vi "Rotronic_monitor.vi"(0 "VISA resource name":refnum<visa-resource-name>="COM1", 1 "baud rate":u32=9600, 2 "data bits":u16=8 min=5 max=8 step=1, 3 "parity":u16(ring) items=["None", "Odd", "Even", "Mark", "Space"], 4 "stop bits":u16(ring)=10 items=["1.0"=10, "1.5"=15, "2.0"=20], 5 "write":bool=TRUE, 6 "read":bool=TRUE, 7 "flow control":u16(ring) items=["None"=0, "XON/XOFF"=1, "RTS/CTS"=2, "DTR/DSR"=4], 8 "string to write":string="*IDN?\r\n") -> (9 "read string":string, 10 "bytes read":u32)   [LabVIEW 2019]
doc: "The Basic Serial Read and Write example performs a Serial Port Read, a Serial Port Write, or a combination of these actions. The user selects the actions (read or write) on the front panel. If both are selected, the VI will write the data first, read data, and then close the VISA session that is opened to the port. This VI will wait until the specified number of bytes is received at the port. Only the number of bytes specified will be read.\n\nINSTRUCTIONS:\n1) Select the serial resource and configuration parameters (baud rate, data bits, parity, stop bits, flow control).\n2) Select the operations to be performed. \n3) Connect the serial port to your device. If no device is available, perform a loopback test by doing one of the following. Short pins 2 and 3 on a RS-232 cable or short pin 4 to pin 8 and pin 5 to pin 9 on a RS-485/422 cable. \n4) Run the VI to see the data read. (The \"read string\" will match the \"string to write\" if a loopback test was performed.)\n\nNote: The parameters set for the serial port must match the parameters of the connected instrument or device. In this example, the bytes to read parameter specifies the number of bytes that the serial port reads. If there were more bytes at the port than the number specified in bytes to read, those bytes would not be read. Also, if you specify to read more bytes than the number of bytes actually read, you might receive a timeout error message.\n\nOn the block diagram, the Configure Serial Port VI sets the configuration parameters. The front panel displays the controls used to configure the basic parameters, such as baud rate, data bits, and parity. Constants configure the other parameters the user probably does not need set. After the VISA Configure Serial Port VI opens the VISA session and configures the port, the VI passes the VISA resource name to other VIs that perform operations on that VISA resource. The VISA Write function sends a command to the serial device and the VISA Read function returns data based on the command. The VISA Close function then closes the reference to the serial device. It is important to close the reference; otherwise communication through with that port through protocols other than VISA might not be possible."
uses:
  <vilib>/Instr/_visa.llb/VISA Configure Serial Port (Instr).vi
panel:
  out "N2 temperature > dew point":bool
  in  "File Path Control":path
  out "Last Line":string[](array[string])
  in  "Quit":bool
  in  "delay before read (ms)":u32=500
  # "Select the serial resource and the operations (Read, Write, or both) to be performed.  If both are selected, the VI will write the data first, read data and then close the VISA session that is opened to the port.  This VI will wait until the specified number of bytes is received at the port. Only the number of bytes specified will be read."
  # "For additional information select File >> VI Properties >> Documentation"
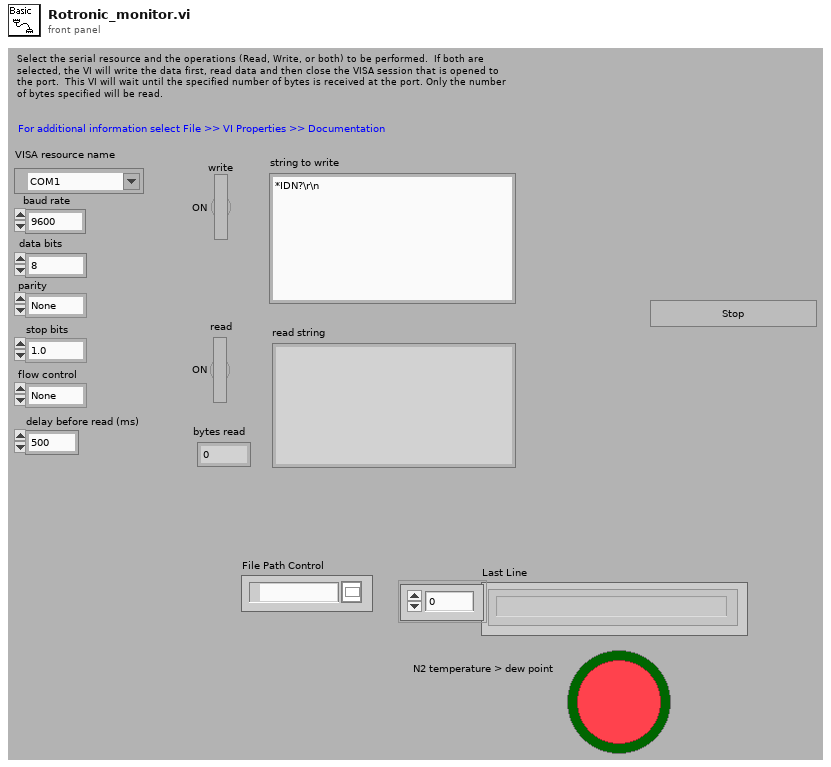
[diagram p1: front panel]
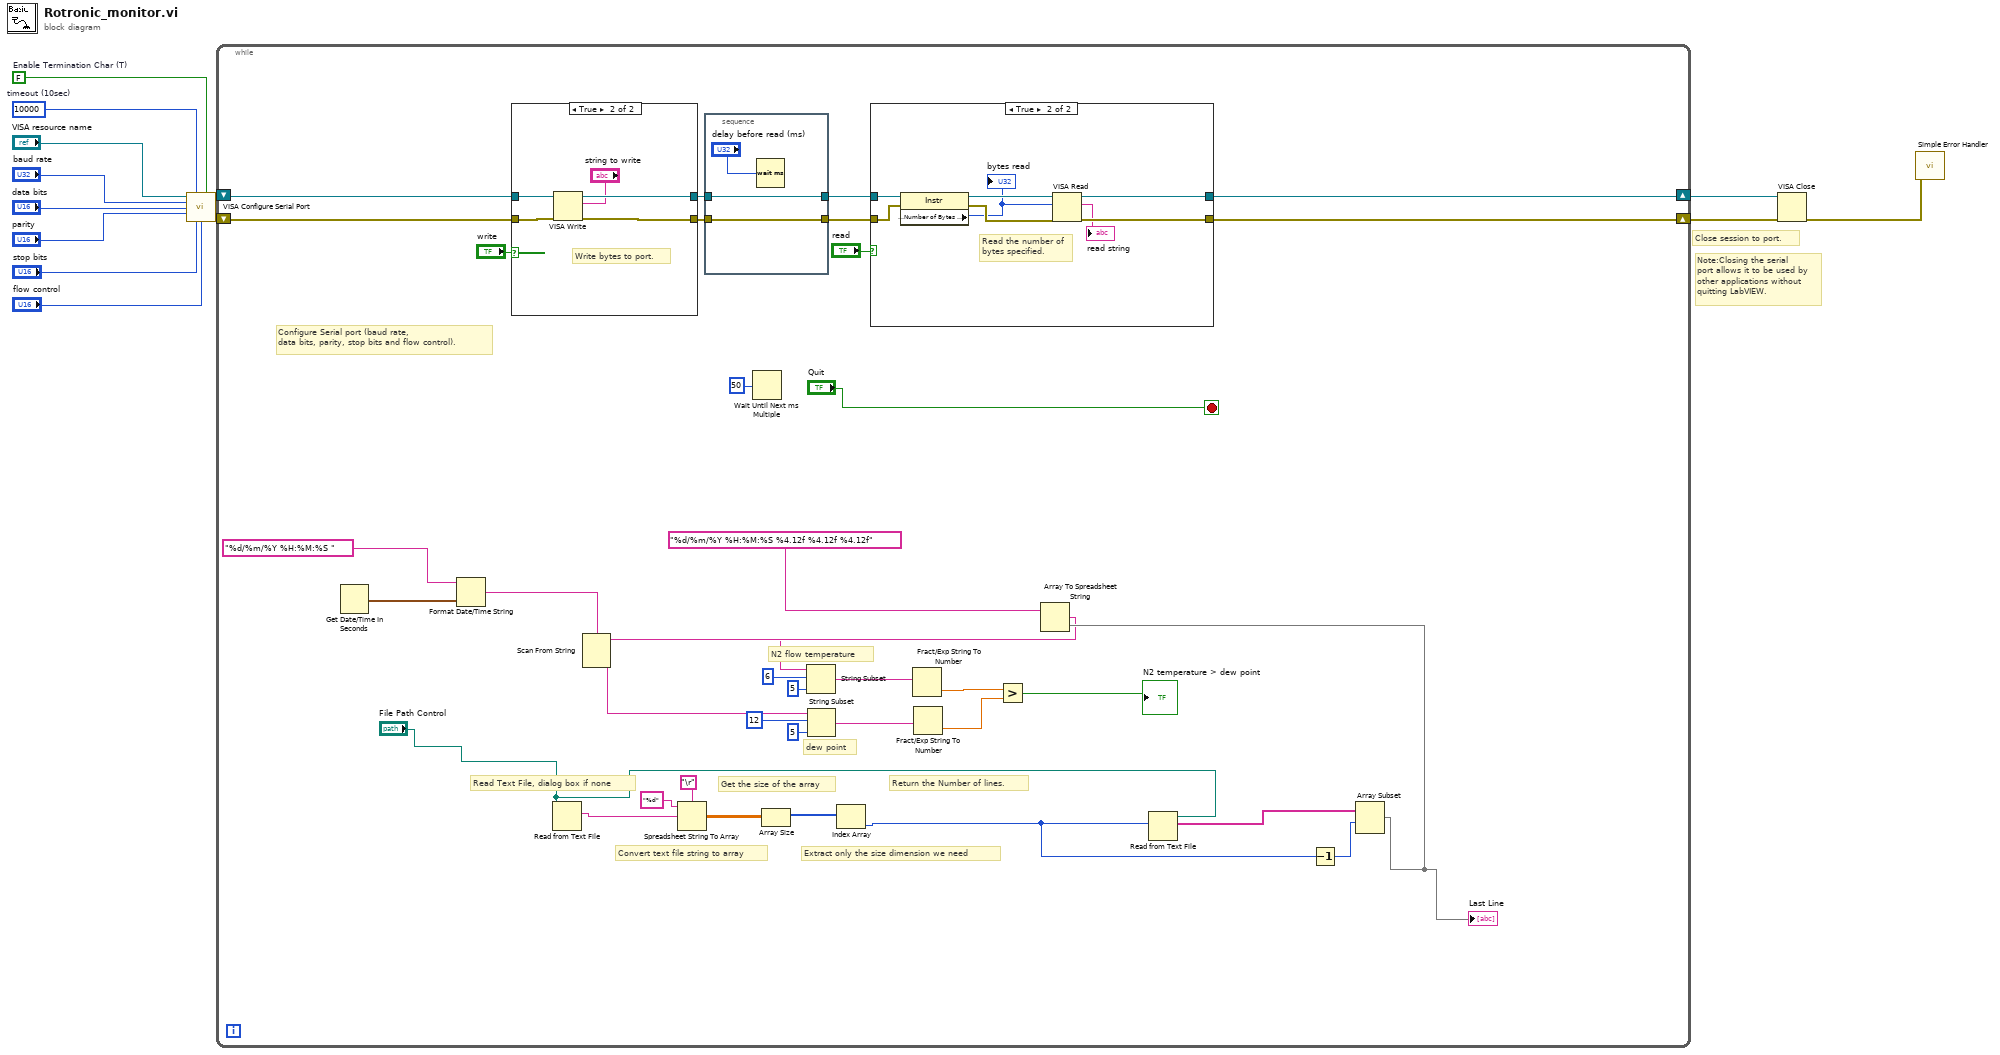
[diagram p0: block diagram]
diagram:
  w4 = FALSE  # Enable Termination Char (T)
  w5 = u32 10000  # timeout (10sec)
  # "Note:Closing the serial port allows it to be used by other applications without\nquitting LabVIEW."
  # "Close session to port."
  n1 = call-poly "VISA Configure Serial Port"("VISA resource name"="VISA resource name", "timeout (10sec)"=w5, "Enable Termination\nChar (T)"=w4, "baud rate (9600)"="baud rate", "data bits (8)"="data bits", "parity (0:none)"="parity", "stop bits (10: 1 bit)"="stop bits", "flow control (0:none)"="flow control") -> ("VISA resource name out"=w10:refnum<visa-resource-name>, "error out"=w11:errorcluster)  [unwired: 6 in]
  n2 = while {
    shift-right: [w47] -> w9
    shift-left: w11 -> [w49]
    shift-right: [w46] -> w8
    shift-left: w10 -> [w48]
    stop <- "Quit" stop-if-true
    # "dew point"
    # "N2 flow temperature"
    # "Convert text file string to array"
    # "Return the Number of lines."
    # "Extract only the size dimension we need"
    # "Get the size of the array"
    # "Read Text File, dialog box if none"
    # "Configure Serial port (baud rate,\ndata bits, parity, stop bits and flow control)."
    n3 = Get Date/Time In Seconds() -> (seconds since 1Jan1904=w38:timestamp)
    n4 = Format Date/Time String(time format string (%c)="%d/%m/%Y %H:%M:%S ", seconds (now)=w38) -> (date/time string=w36:string)  [unwired: 1 in]
    n5 = case shown="True" "write" {
      tunnel: [w55 w60] -> w44
      tunnel: w48 -> [w54 w59]
      tunnel: w49 -> [w55 w58]
      tunnel: [w54 w57] -> w42
      frame False {
      }
      frame True {
        # "Write bytes to port."
        n6 = VISA Write(VISA resource name=w59, write buffer="string to write", error in (no error)=w58) -> (VISA resource name out=w57:refnum<visa-resource-name>, error out=w60:errorcluster)  [unwired: 1 out]
      }
    }
    n7 = Read from Text File(file (use dialog)="File Path Control") -> (text=w31:string)  [unwired: 1 in, 5 out]
    n8 = Spreadsheet String To Array(delimiter (Tab)="\r", format string="%d", spreadsheet string=w31) -> (array=w33:dbl[][])  [unwired: 1 out]
    n9 = stacked-sequence {
      tunnel: w44 -> [w53]
      tunnel: [w53] -> w43
      tunnel: w42 -> [w52]
      tunnel: [w52] -> w41
      frame #0 {
        n10 = Wait (ms)(milliseconds to wait="delay before read (ms)") -> ()  [unwired: 1 out]
      }
    }
    n11 = Wait Until Next ms Multiple(millisecond multiple=u32 50) -> ()  [unwired: 1 out]
    n12 = Array Size(array=w33) -> (size(s)=w32:i32[])
    n13 = Index Array(array=w32) -> (element=w28:i32)  [unwired: 1 in]
    n14 = case shown="True" "read" {
      tunnel: w43 -> [w62 w66]
      tunnel: [w62 w70] -> w47
      tunnel: [w61 w69] -> w46
      tunnel: w41 -> [w61 w68]
      frame False {
      }
      frame True {
        # "Read the number of bytes specified."
        n15 = property class="Instr"(reference=w68, error in=w66) -> (reference out=w67:refnum<visa-resource-name>, error out=w65:errorcluster, "Serial Settings:Number of Bytes at Serial Port"=w64:u32)
        "bytes read" <- w64
        n16 = VISA Read(VISA resource name=w67, byte count=w64, error in (no error)=w65) -> (VISA resource name out=w69:refnum<visa-resource-name>, read buffer=→"read string":string, error out=w70:errorcluster)  [unwired: 1 out]
      }
    }
    n17 = Read from Text File(file (use dialog)="File Path Control", count=w28) -> (text=w27:string[])  [unwired: 1 in, 4 out]
    n18 = Decrement(x=w28) -> (x-1=w30:i32)
    n19 = Array Subset(array=w27, index=w30) -> (w26:string[])  [unwired: 1 in]
    "Last Line" <- w26
    n20 = Array To Spreadsheet String(array=w26, 3:"%d/%m/%Y %H:%M:%S %4.12f %4.12f %4.12f" ("time format string (%c)")) -> (spreadsheet string=w24:string)  [unwired: 1 in]
    n21 = Scan From String(format string=w36, input string=w24) -> (remaining string=w21:string)  [unwired: 4 in, 2 out]
    n22 = String Subset(string=w21, offset (0)=6, length (rest)=5 ("length (rest)")) -> (substring=w18:string)
    n23 = String Subset(string=w21, offset (0)=12, length (rest)=5 ("length (rest)")) -> (substring=w17:string)
    n24 = Fract/Exp String To Number(string=w18) -> (number=w16:dbl)  [unwired: 3 in, 1 out]
    n25 = Fract/Exp String To Number(string=w17) -> (number=w15:dbl)  [unwired: 3 in, 1 out]
    n26 = Greater?(x=w16, y=w15) -> (0:→"N2 temperature > dew point":bool)
  }
  n27 = VISA Close(VISA resource name=w8, error in (no error)=w9) -> (error out=w7:errorcluster)
  n28 = call <vilib>:"Simple Error Handler.vi"("error in (no error)"=w7) -> ()  [unwired: 4 in, 5 out]
